vi "example_relativePlacement.vi"() -> ()   [LabVIEW 2023]
doc: "This example shows how to use the Relative Placement VIs to place a 'movingObject' in a specific position relative to an 'anchorObject'."
uses:
  <vilib>/numeric/Random Number (Range) U64.vi
  <vilib>/numeric/sub_Random U32.vi
panel:
  in  "spacing[pixels]":u16
  in  "placeBottom":bool
  in  "placeAbove":bool
  in  "useControlBodyOnly":bool=TRUE caption="Use Ctrl Body Only\n(=ignore labels \n& captions)"
  in  "stop":bool
  in  "placeRightOf":bool
  in  "placeLeftOf":bool
  in  "shuffle":bool
  in  "anchorObject":string
  in  "movingObject":dbl
  # "Instruction:\n1. Press Shuffle button to place the target objects randomly.\n2. Press the Alignment button you prefer."
  # "Relative placement"
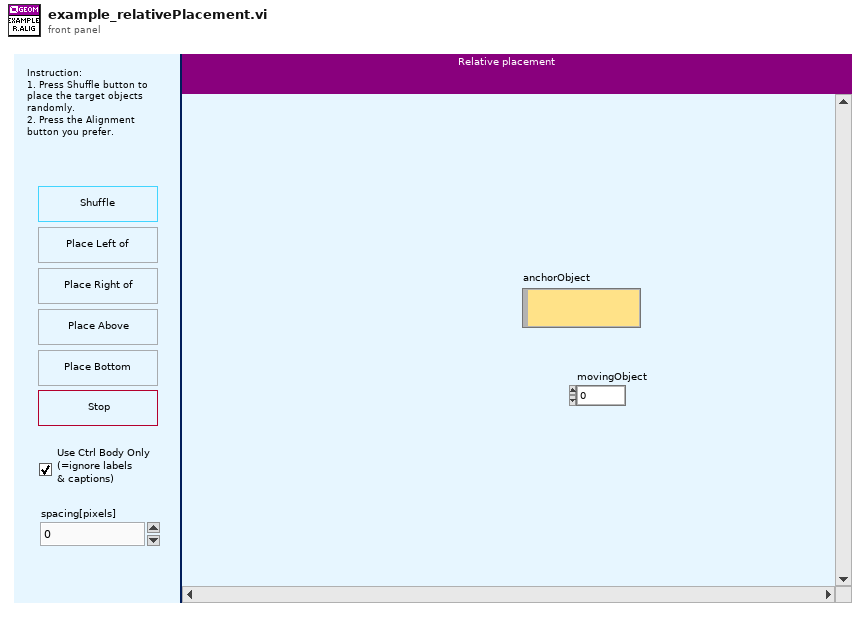
[diagram p1: front panel]
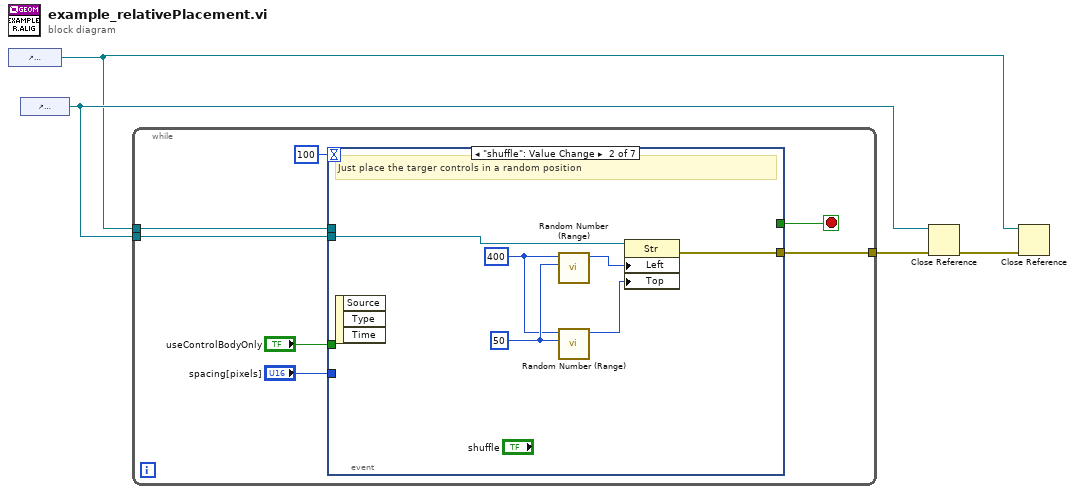
[diagram p0: block diagram]
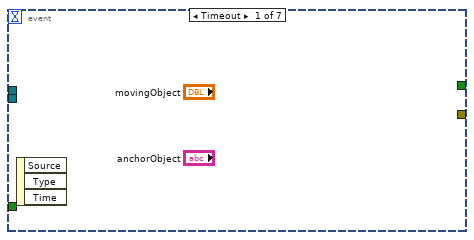
[diagram p2: hidden frame]
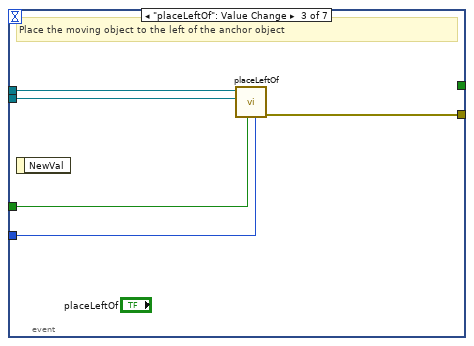
[diagram p3: hidden frame]
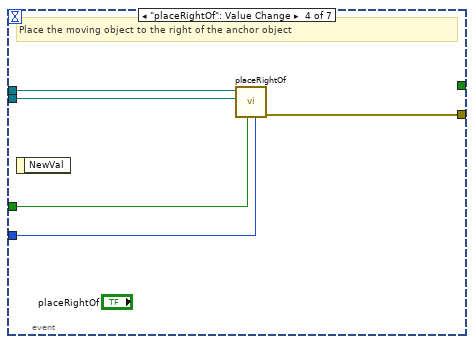
[diagram p4: hidden frame]
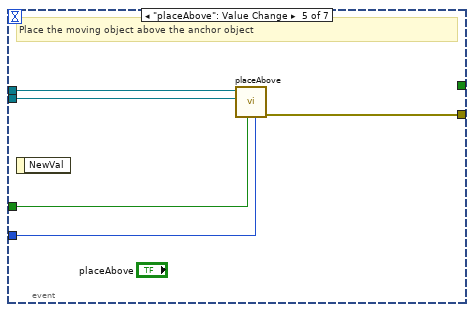
[diagram p5: hidden frame]
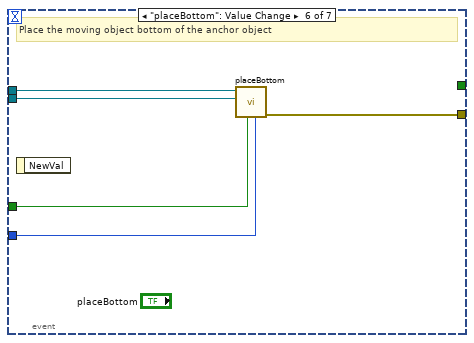
[diagram p6: hidden frame]
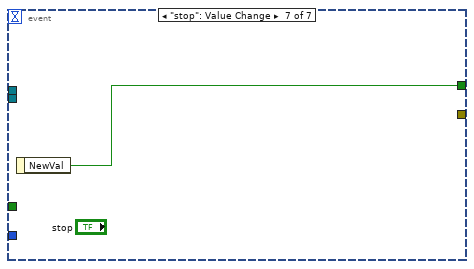
[diagram p7: hidden frame]
diagram:
  n1 = control-ref of="movingObject"() -> (w1:refnum<vi>)
  n2 = control-ref of="anchorObject"() -> (w2:refnum<vi>)
  n3 = while {
    tunnel: w2 -> [w10]
    tunnel: [w9] -> w4
    tunnel: w1 -> [w7]
    stop <- w11 stop-if-true
    n4 = event shown="[1] \"shuffle\": Value Change" {
      selector: _ -> [_ _ _ _ _ _ _]
      dyn-events: _ -> [_ _ _ _ _ _ _]
      timeout: 100 -> [_ _ _ _ _ _ _]
      tunnel: [_ _ _ _ _ _ w38] -> w11
      tunnel: w10 -> [_ w17 w20 w25 w30 w35 _]
      tunnel: [_ w16 w21 w26 w31 w36 _] -> w9
      tunnel: "useControlBodyOnly" -> [_ _ w22 w27 w32 w37 _]
      tunnel: w7 -> [_ _ w19 w24 w29 w34 _]
      tunnel: "spacing[pixels]" -> [_ _ w18 w23 w28 w33 _]
      event Timeout {
        n5 = event-data() -> ()  [unwired: 1 in, 3 out]
      }
      event "shuffle": Value Change {
        w12 = u64 400 ("lower bound (0)")
        w13 = u64 50 ("lower bound (0)")
        # "Just place the targer controls in a random position"
        n6 = event-data() -> ()  [unwired: 1 in, 3 out]
        n7 = call-poly <vilib>:"Random Number (Range).vi"("lower bound (0)"=w13, "upper bound (100)"=w12) -> ("number"=w15:u64)  [unwired: 9 in]
        n8 = call-poly <vilib>:"Random Number (Range).vi"("lower bound (0)"=w13, "upper bound (100)"=w12) -> ("number"=w14:u64)  [unwired: 9 in]
        n9 = property class="Str"(reference=w17, "Left"=w15, "Top"=w14) -> (error out=w16:errorcluster)  [unwired: 1 in, 1 out]
      }
      event "placeLeftOf": Value Change {
        # "Place the moving object to the left of the anchor object"
        n10 = event-data() -> ()  [unwired: 1 in, 1 out]
        n11 = call "placeLeftOf.vi"("spacing[pixel]"=w18, "useControlBodyOnly"=w22, "anchorObject"=w20, "movingObject"=w19) -> ("error out"=w21:errorcluster)  [unwired: 5 in, 2 out]
      }
      event "placeRightOf": Value Change {
        # "Place the moving object to the right of the anchor object"
        n12 = event-data() -> ()  [unwired: 1 in, 1 out]
        n13 = call "placeRightOf.vi"("spacing[pixel]"=w23, "useControlBodyOnly"=w27, "anchorObject"=w25, "movingObject"=w24) -> ("error out"=w26:errorcluster)  [unwired: 5 in, 2 out]
      }
      event "placeAbove": Value Change {
        # "Place the moving object above the anchor object"
        n14 = event-data() -> ()  [unwired: 1 in, 1 out]
        n15 = call "placeAbove.vi"("spacing[pixel]"=w28, "useControlBodyOnly"=w32, "anchorObject"=w30, "movingObject"=w29) -> ("error out"=w31:errorcluster)  [unwired: 5 in, 2 out]
      }
      event "placeBottom": Value Change {
        # "Place the moving object bottom of the anchor object"
        n16 = event-data() -> ()  [unwired: 1 in, 1 out]
        n17 = call "placeBottom.vi"("spacing[pixel]"=w33, "useControlBodyOnly"=w37, "anchorObject"=w35, "movingObject"=w34) -> ("error out"=w36:errorcluster)  [unwired: 5 in, 2 out]
      }
      event "stop": Value Change {
        n18 = event-data() -> ("NewVal"=w38:bool)  [unwired: 1 in]
      }
    }
  }
  n19 = Close Reference(reference=w2, error in (no error)=w4) -> (error out=w3:errorcluster)
  n20 = Close Reference(reference=w1, error in (no error)=w3) -> ()  [unwired: 1 out]
